vi "SPL Calibration.vi"() -> ()   [LabVIEW 2013]
panel:
  in  "Gain":dbl(slide) min=-30.0 max=50.0 scale=-30.0..30.0
  out "SPL":dbl
  out "Acoustics":dynamicdata(graph)
  in  "stop (F)":bool
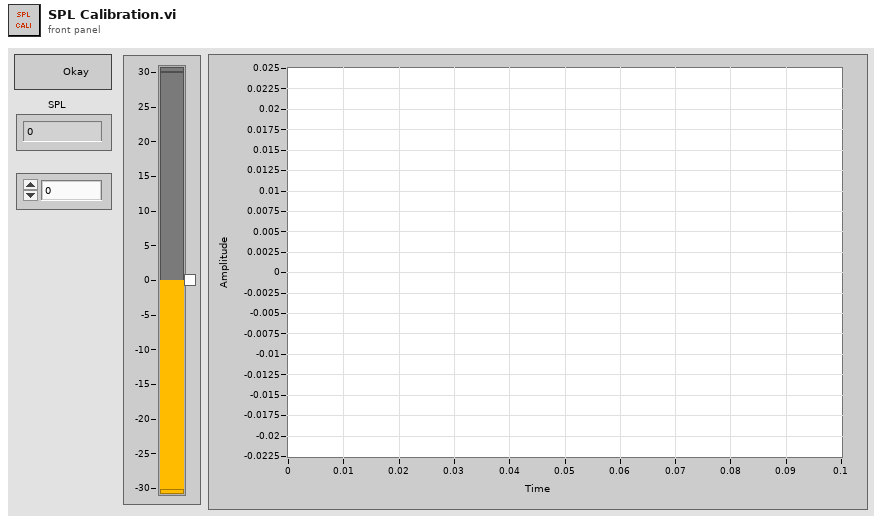
[diagram p1: front panel]
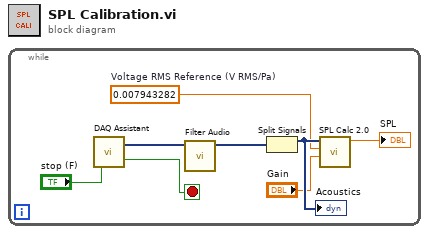
[diagram p0: block diagram]
diagram:
  n1 = while {
    stop <- w7 stop-if-true
    w5 = 0.007943282  # Voltage RMS Reference (V RMS/Pa)
    n2 = call "DAQ Assistant"("stop (F)"="stop (F)") -> ("data"=w2:dynamicdata, "stopped"=w7:bool)  [unwired: 15 in, 2 out]
    n3 = call "Filter Audio"("Signal"=w2) -> ("Filtered Signal"=w1:dynamicdata)  [unwired: 9 in, 1 out]
    n4 = Split Signals(w1) -> (w6:dynamicdata)  [unwired: 2 in, 1 out]
    "Acoustics" <- w6
    n5 = call "SPL Calc 2.0.vi"("Gain"="Gain", "Voltage RMS Reference (V RMS/Pa)"=w5, "Dynamic Data"=w6) -> ("SPL"=→"SPL":dbl)  [unwired: 8 in]
  }
